vi "Byte Buffer.Mapping.Get Largest Count.vi"(11 "mappings":T1[](array[typedef])) -> (2 "largest count":i32, 3 "mappings dup":T1[](array[typedef]))   [LabVIEW 2016, in "VeriStand Data.lvlib" / "Byte Buffer.lvclass"]
uses:
  Byte Buffer.lvclass
  Byte Buffer.Mapping.ctl
  Typedefs/Typedefs.Data Types.ctl
  VeriStand Data.lvlib
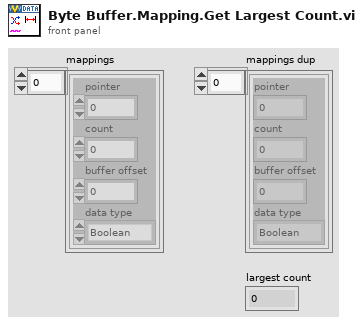
[diagram p1: front panel]
types:
  T1 = typedef "VeriStand Data.lvlib/Byte Buffer.lvclass/Byte Buffer.Mapping.ctl" = cluster{"pointer":u64, "count":i32, "buffer offset":i32, "data type":T2}
  T2 = typedef "VeriStand Data.lvlib/Typedefs.Data Types.ctl" = enum16{"Boolean", "Single", "Double", "I8", "I16", "I32", "I64", "U8", "U16", "U32", "U64"}
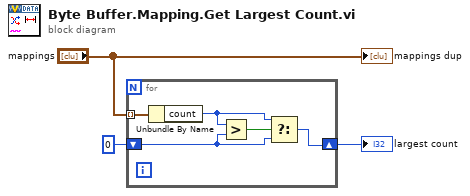
[diagram p0: block diagram]
diagram:
  n1 = for {
    tunnel: "mappings" -> [w8] mode=indexing
    shift-right: [w7] -> w2
    shift-left: 0 -> [w6]
    n2 = Unbundle By Name(w8) -> ("count"=w4:i32)
    n3 = Greater?(x=w4, y=w6) -> (0:w5:bool)
    n4 = Select(t=w4, s=w5, f=w6) -> (s? t:f=w7:i32)
  }
  "largest count" <- w2
  "mappings dup" <- "mappings"
